vi "Thermistor volts to temperature.vi"(1 "V2 (V)":dbl=1.24) -> (0 "Temperature (degC)":dbl=25.0)   [LabVIEW 2011]
panel:
  in  "T0 (K)":dbl=298.15
  in  "R1(T0) (ohms)":dbl=100000.0
  in  "R2 (ohms)":dbl=100000.0
  in  "B (K)":dbl=4334.0
  in  "Vs (V)":dbl=2.48
  # "Paul Nathan 26/07/2012"
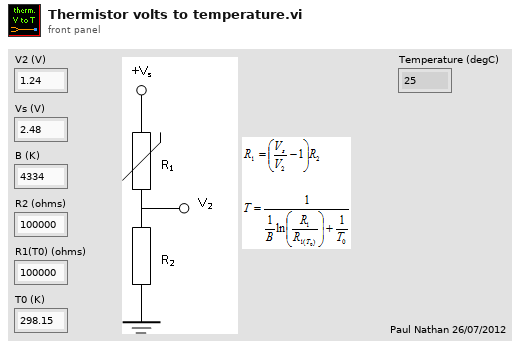
[diagram p1: front panel]
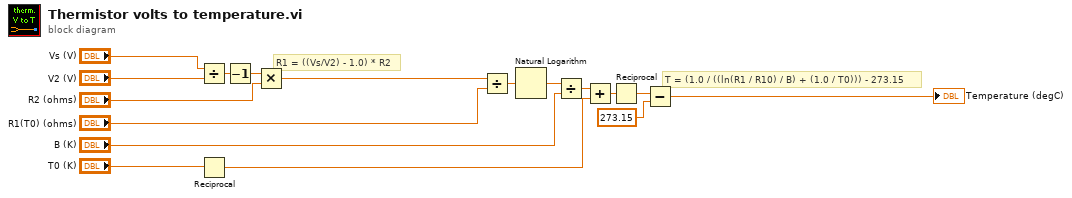
[diagram p0: block diagram]
diagram:
  # "T = (1.0 / ((ln(R1 / R10) / B) + (1.0 / T0))) - 273.15"
  # "R1 = ((Vs/V2) - 1.0) * R2"
  n1 = Divide(x="Vs (V)", y="V2 (V)") -> (x/y=w15:dbl)
  n2 = Reciprocal(x="T0 (K)") -> (1/x=w8:dbl)
  n3 = Decrement(x=w15) -> (x-1=w13:dbl)
  n4 = Multiply(x=w13, y="R2 (ohms)") -> (x*y=w12:dbl)
  n5 = Divide(x=w12, y="R1(T0) (ohms)") -> (x/y=w6:dbl)
  n6 = Natural Logarithm(1:w6) -> (0:w5:dbl)
  n7 = Divide(x=w5, y="B (K)") -> (x/y=w4:dbl)
  n8 = Add(x=w4, y=w8) -> (x+y=w3:dbl)
  n9 = Reciprocal(x=w3) -> (1/x=w2:dbl)
  n10 = Subtract(x=w2, y=273.15) -> (x-y=→"Temperature (degC)":dbl)
